vi "Read Byte.vi"(8 "error in (no error)":errorcluster, 10 "IOCON.BANK = 0 Reg Addresses":T2, 11 "Chip Address (A2 A1 A0)":T3 max=7) -> (0 "error out":errorcluster, 3 "SPI Command":T1)   [LabVIEW 2014, in "MCP23S17.lvlib"]
doc: "Reads a byte of data of the desired register."
uses:
  MCP23S17.lvlib
  Chip Address.ctl
  IOCON BANK 0 Reg Addresses.ctl
  SPI Command.ctl
  OPCODE.ctl
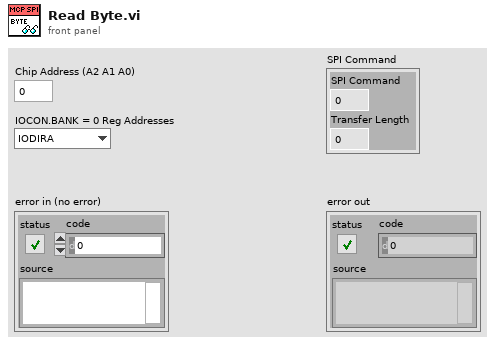
[diagram p1: front panel]
types:
  T1 = typedef "MCP23S17.lvlib/SPI Command.ctl" = cluster{"SPI Command":u32, "Transfer Length":u8}
  T2 = typedef "MCP23S17.lvlib/IOCON BANK 0 Reg Addresses.ctl" = enum8{"IODIRA", "IODIRB", "IPOLA", "IPOLB", "GPINTENA", "GPINTENB", "DEFVALA", "DEFVALB", "INTCONA", "INTCONB", "IOCONA", "IOCONB", "GPPUA", "GPPUB", "INTFA", "INTFB", "INTCAPA", "INTCAPB", "GPIOA", "GPIOB", "OLATA", "OLATB"}
  T3 = typedef "MCP23S17.lvlib/Chip Address.ctl" = u8
  T4 = typedef "MCP23S17.lvlib/OPCODE.ctl" = u8
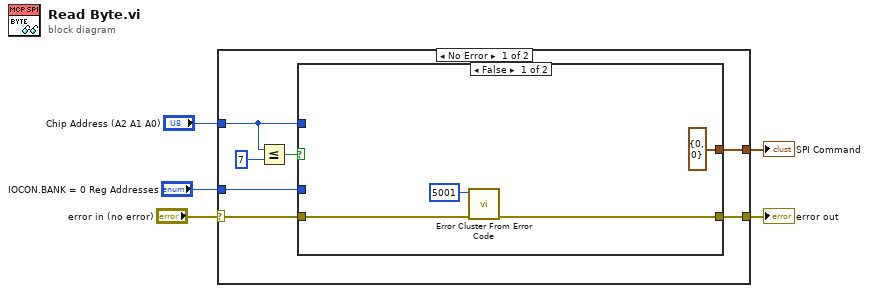
[diagram p0: block diagram]
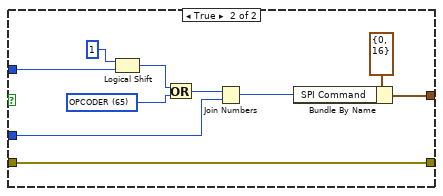
[diagram p2: hidden frame]
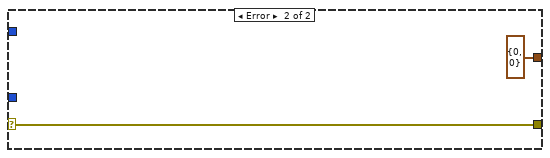
[diagram p3: hidden frame]
diagram:
  n1 = case shown="No Error" "error in (no error)" {
    selector: "error in (no error)" -> [w8 w28]
    tunnel: "IOCON.BANK = 0 Reg Addresses" -> [w12 _]
    tunnel: "Chip Address (A2 A1 A0)" -> [w11 _]
    tunnel: [w7 w28] -> w2
    tunnel: [w6 T1 {"SPI Command"=0, "Transfer Length"=0} ("SPI Command")] -> w1
    frame No Error {
      n2 = Less Or Equal?(x=w11, y=T3 7) -> (x <= y?=w9:bool)
      n3 = case shown="False" w9 {
        tunnel: w11 -> [_ w26]
        tunnel: w12 -> [_ w21]
        tunnel: w8 -> [w16 w20]
        tunnel: [w15 w20] -> w7
        tunnel: [T1 {"SPI Command"=0, "Transfer Length"=0} ("SPI Command") w17] -> w6
        frame False {
          n4 = call <vilib>:"Error Cluster From Error Code.vi"("error in (no error)"=w16, "error code (0)"=5001) -> ("error out"=w15:errorcluster)  [unwired: 7 in]
        }
        frame True {
          w23 = T4 65 items=["OPCODEW"=64, "OPCODER"=65, "ADDR_ENABLE"=8] ("OPCODE")
          n5 = Logical Shift(y=i16 1, x=w26) -> (x << y=w24:T3)
          n6 = Or(x=w24, y=w23) -> (x .or. y?=w22:T3)
          n7 = Join Numbers(hi=w22, lo=w21) -> ((hi.lo)=w18:u16)
          n8 = Bundle By Name(cluster=T1 {"SPI Command"=0, "Transfer Length"=16} ("SPI Command"), "SPI Command"=w18) -> (w17:T1)
        }
      }
    }
    frame Error {
    }
  }
  "error out" <- w2
  "SPI Command" <- w1
